vi "IOScan_UIStrings.vi"() -> ()   [LabVIEW 2016]
panel:
  in  "Scan Warning":string="警告：将扫描周期设置为低于%d %s可能导致系统不稳定。对于时序故障，请监控终端上的NI扫描引擎故障。" caption="扫描警告"
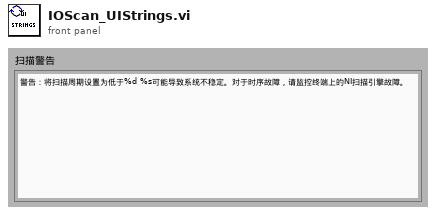
[diagram p1: front panel]
diagram:
